vi "New Session SetUp.vi"(8 "error in (no error)":errorcluster, 10 "Stop Refnum":refnum<vi>, 11 "Fluke Hydra 2625A in":refnum<class "Fluke Hydra 2625A.lvclass">) -> (0 "error out":errorcluster, 3 "output cluster":refnum<class "Fluke Hydra 2625A.lvclass">)   [LabVIEW 2014, in "Generic Data Acquisition.lvlib" / "Fluke Hydra.lvlib" / "Fluke Hydra 2625A.lvclass"]
uses:
  Fluke Hydra 2625A.lvclass
  Unit Measurement.ctl
  Generic Data Acquisition.lvclass
  <instrlib>/Fluke 2625A/Fluke 2625A.lvlib
  Subpanel Insertion/Subpanel Inserter.lvclass
panel:
  in  "Boolean 2":bool=TRUE
  in  "Stop Button":bool
  out "ID":string
  out "Boolean":bool
  out "i":i32
  in  "Array":T1[](array[typedef]) {"Thermocouple Type (0: J) 2" items=["J", "K", "E", "T", "N", "R", "S", "B", "C"]; "Channel" min=0 max=20 step=1; "Function (5: Temp)" items=["OFF", "Vdc", "Vac", "Ohms", "Freq", "TEMP"]}
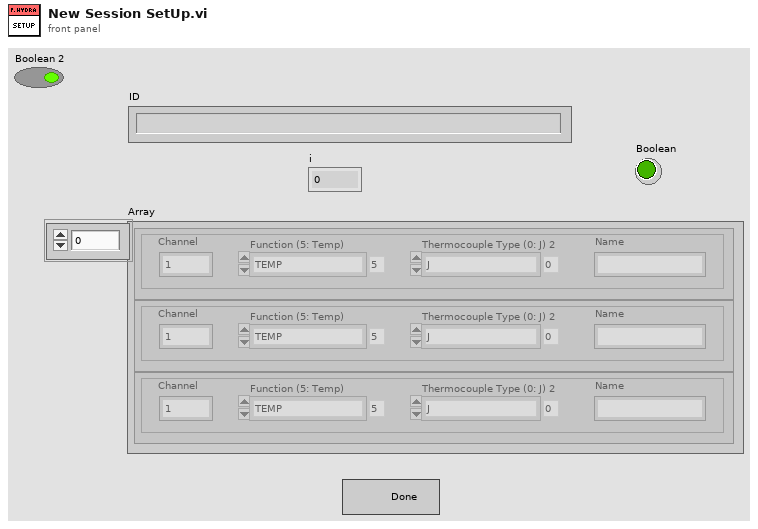
[diagram p1: front panel]
types:
  T1 = typedef "Unit Measurement.ctl" = cluster{"Function (5: Temp)":u16, "Channel":i8, "Thermocouple Type (0: J) 2":u16, "Name":string}
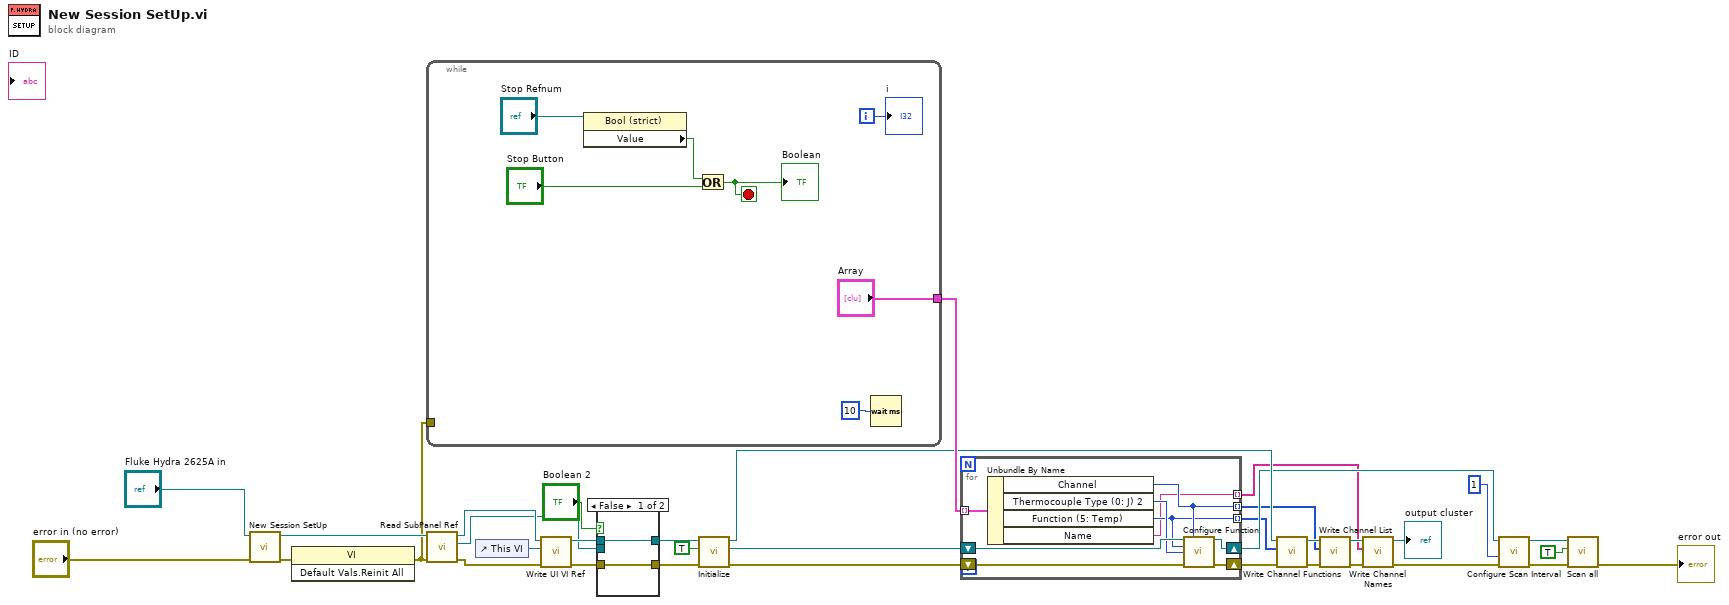
[diagram p0: block diagram]
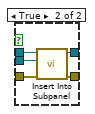
[diagram p2: hidden frame]
diagram:
  n1 = call-parent "New Session SetUp.vi"("error in (no error)"="error in (no error)", "Generic Data Acquisition in"="Fluke Hydra 2625A in") -> ("error out"=w14:errorcluster, "output cluster"=w13:refnum<class "Fluke Hydra 2625A.lvclass">)  [unwired: 8 in]
  n2 = invoke class="VI" method="Default Vals.Reinit All"(error in=w14) -> (error out=w10:errorcluster)  [unwired: 2 in, 2 out]
  n3 = while {
    tunnel: ["Array"] -> w35
    tunnel: w10 -> [_]
    i -> [w41]
    stop <- w36 stop-if-true
    n4 = property class="Bool (strict)"(reference="Stop Refnum") -> ("Value"=w37:bool)  [unwired: 1 in, 2 out]
    n5 = Or(x=w37, y="Stop Button") -> (x .or. y?=w36:bool)
    "Boolean" <- w36
    n6 = Wait (ms)(milliseconds to wait=u32 10) -> ()  [unwired: 1 out]
    "i" <- w41
  }
  n7 = call-dynamic "Read SubPanel Ref.vi"("error in (no error)"=w10, "Subpanel Inserter in"=w13) -> ("error out"=w11:errorcluster, "SubPanel Ref"=w5:refnum<vi>, "Subpanel Inserter out"=w12:refnum<class "Fluke Hydra 2625A.lvclass">)  [unwired: 7 in]
  n8 = control-ref of="This VI"() -> (w30:refnum<vi>)
  n9 = call-dynamic "Write UI VI Ref.vi"("error in (no error)"=w11, "UI VI Ref"=w30, "Subpanel Inserter in"=w12) -> ("error out"=w8:errorcluster, "Subpanel Inserter out"=w9:refnum<class "Fluke Hydra 2625A.lvclass">)  [unwired: 7 in]
  n10 = case shown="False" "Boolean 2" {
    tunnel: w9 -> [w44 w49]
    tunnel: w8 -> [w43 w48]
    tunnel: [w44 w47] -> w7
    tunnel: [w43 w46] -> w6
    tunnel: w5 -> [_ w45]
    frame False {
    }
    frame True {
      n11 = call "Insert Into Subpanel.vi"("Error In"=w48, "SubPanel Ref"=w45, "Subpanel Inserter"=w49) -> ("error out"=w46:errorcluster, "Subpanel Inserter"=w47:refnum<class "Fluke Hydra 2625A.lvclass">)  [unwired: 7 in]
    }
  }
  n12 = call-dynamic "Initialize.vi"("error in (no error)"=w6, "Reset"=TRUE, "Fluke Hydra 2625A in"=w7) -> ("error out"=w32:errorcluster, "VISA resource name"=w34:refnum<visa-resource-name>, "Fluke Hydra 2625A out"=w33:refnum<class "Fluke Hydra 2625A.lvclass">)  [unwired: 6 in]
  n13 = for {
    tunnel: w35 -> [w58] mode=indexing
    tunnel: [w56] -> w21 mode=indexing
    shift-right: [w54] -> w17
    shift-left: w32 -> [w55]
    shift-right: [w53] -> w26
    shift-left: w34 -> [w57]
    tunnel: [w51] -> w18 mode=indexing
    tunnel: [w50] -> w22 mode=indexing
    n14 = Unbundle By Name(w58) -> ("Channel"=w56:i8, "Thermocouple Type (0: J) 2"=w52:u16, "Function (5: Temp)"=w51:u16, "Name"=w50:string)
    n15 = call <instrlib>:"Configure Function.vi"("VISA Resource Name In"=w57, "Channel In"=w56, "Function (5: Temp) In"=w51, "Thermocouple Type (0: J) In"=w52, "Error In"=w55) -> ("VISA Resource Name Out"=w53:refnum<visa-resource-name>, "Error Out"=w54:errorcluster)  [unwired: 8 in, 1 out]
  }
  n16 = call-dynamic "Write Channel Functions.vi"("error in (no error)"=w17, "Channel Functions"=w18, "Generic Data Acquisition in"=w33) -> ("error out"=w19:errorcluster, "Generic Data Acquisition out"=w24:refnum<class "Fluke Hydra 2625A.lvclass">)  [unwired: 7 in]
  n17 = call-dynamic "Write Channel List.vi"("error in (no error)"=w19, "Channel List"=w21, "Generic Data Acquisition in"=w24) -> ("error out"=w20:errorcluster, "Generic Data Acquisition out"=w23:refnum<class "Fluke Hydra 2625A.lvclass">)  [unwired: 7 in]
  n18 = call-dynamic "Write Channel Names.vi"("error in (no error)"=w20, "Channel Names"=w22, "Generic Data Acquisition in"=w23) -> ("error out"=w16:errorcluster, "Generic Data Acquisition out"=→"output cluster":refnum<class "Fluke Hydra 2625A.lvclass">)  [unwired: 7 in]
  n19 = call <instrlib>:"Configure Scan Interval.vi"("Error In"=w16, "Seconds In"=i8 1, "VISA Resource Name In"=w26) -> ("Error Out"=w27:errorcluster, "VISA Resource Name Out"=w25:refnum<visa-resource-name>)  [unwired: 7 in]
  n20 = call <instrlib>:"Scan all.vi"("Error In"=w27, "Start/Stop In"=TRUE, "VISA Resource Name In"=w25) -> ("Error Out"=→"error out":errorcluster)  [unwired: 6 in, 2 out]
